vi "Non Delay Scheduler For Tardiness.vi"(8 "Number of  Jobs":i32=4, 9 "Number of Machines":i32=4, 10 "Processing Times":u16[][](array[numeric])=[[34, 15, 38, 95], [2, 89, 19, 7], [54, 70, 28, 34], [61, 9, 87, 29]], 11 "Schedule":u16[](array[numeric])=[12, 0, 7, 2, 6, 3, 13, 5, 1, 4, 14, 11, 10, 15, 8, 9]) -> (0 "Scheduled Jobs Order":u16[](array[numeric]), 1 "Job Completion Times":u16[](array[numeric]), 2 "Completion Times":u16[][](array[numeric]), 3 "Start Times":u16[][](array[numeric]), 4 "Machine Completion Times":u16[](array[numeric]))   [LabVIEW 2013, in "Scheduler.lvclass"]
uses:
  Scheduler.lvclass
  Priority Rule for ND Tardiness Engine.ctl
panel:
  out "Indices":i32[](array[numeric])
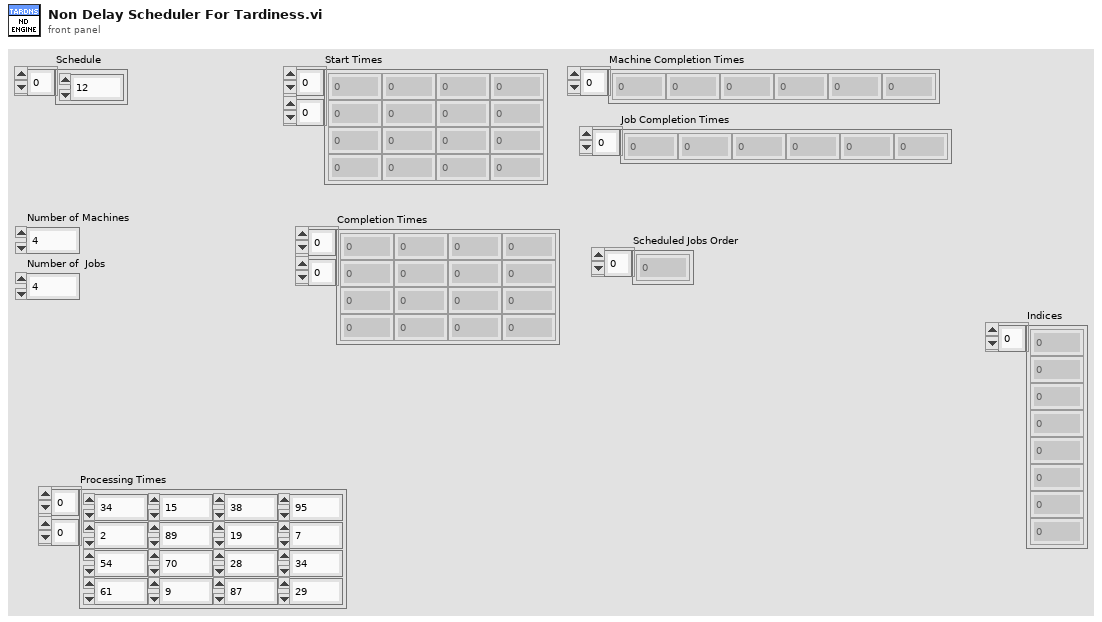
[diagram p1: front panel]
types:
  T1 = typedef "Scheduler.lvclass/Priority Rule for ND Tardiness Engine.ctl" = enum16{"SPT", "MST", "MDD"}
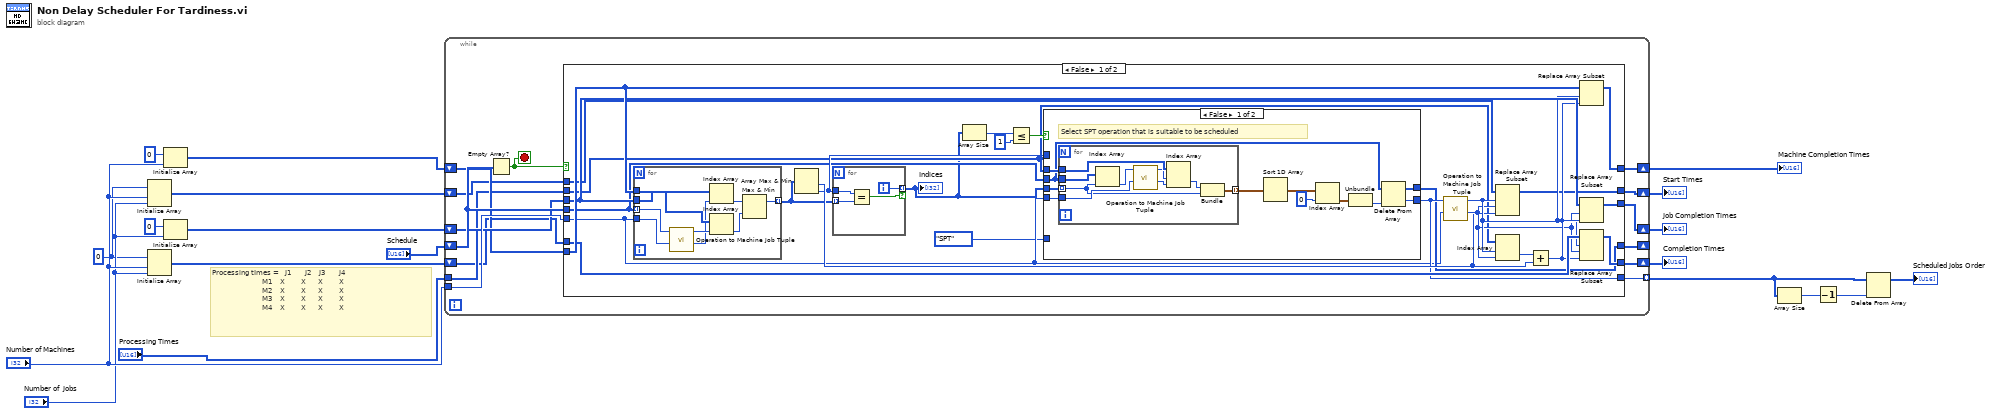
[diagram p0: block diagram]
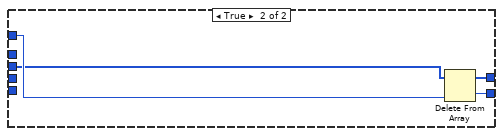
[diagram p2: hidden frame]
diagram:
  w3 = u16 0 ("element")
  # "Processing tImes =   J1       J2    J3       J4   \n                         M1    X        X      X        X\n                         M2    X        X      X        X\n                         M3    X        X      X        X\n                         M4    X        X      X        X"
  n1 = Initialize Array(w3, "Number of Machines", "Number of  Jobs") -> (w2:u16[][])
  n2 = Initialize Array(w3, "Number of Machines", "Number of  Jobs") -> (w14:u16[][])
  n3 = Initialize Array(u16 0 ("element"), "Number of Machines") -> (w16:u16[])
  n4 = Initialize Array(u16 0 ("element"), "Number of  Jobs") -> (w17:u16[])
  n5 = while {
    shift-right: [w25] -> _
    shift-left: "Schedule" -> [w32]
    tunnel: "Number of Machines" -> [w31]
    shift-right: [w28] -> w12
    shift-left: w17 -> [w30]
    shift-right: [w27] -> w11
    shift-left: w16 -> [w29]
    shift-right: [w23] -> w13
    shift-left: w14 -> [w24]
    tunnel: "Processing Times" -> [w26]
    tunnel: [w22] -> w9 mode=indexing
    shift-right: [w20] -> w1
    shift-left: w2 -> [w21]
    stop <- w33 stop-if-true
    n6 = Empty Array?(array=w32) -> (empty?=w33:bool)
    n7 = case shown="False" w33 {
      tunnel: w32 -> [w40 w98]
      tunnel: w31 -> [w35 _]
      tunnel: w30 -> [w57 w100]
      tunnel: w29 -> [w58 w99]
      tunnel: [w56 w100] -> w28
      tunnel: [w55 w99] -> w27
      tunnel: w26 -> [w37 _]
      tunnel: [w38 w98] -> w25
      tunnel: w24 -> [w54 w97]
      tunnel: [w53 w97] -> w23
      tunnel: [w39 _] -> w22
      tunnel: w21 -> [w50 w96]
      tunnel: [w46 w96] -> w20
      frame False {
        n8 = for {
          tunnel: w40 -> [w95] mode=indexing
          tunnel: w35 -> [w94]
          tunnel: w57 -> [w91]
          tunnel: w58 -> [w93]
          tunnel: [w87] -> w45 mode=indexing
          n9 = call "Operation to Machine Job Tuple.vi"("Number of Machines"=w94, "Operation Number"=w95) -> ("Job No"=w90:i32, "Machine No"=w92:i32)  [unwired: 8 in]
          n10 = Index Array(array=w91, index=w90) -> (element=w89:u16)
          n11 = Index Array(array=w93, index=w92) -> (element=w88:u16)
          n12 = Max & Min(x=w89, y=w88) -> (max(x,y)=w87:u16)  [unwired: 1 out]
        }
        n13 = Array Max & Min(array=w45) -> (min value=w47:u16, min index (indices)=w41:i32)  [unwired: 2 out]
        n14 = for {
          tunnel: w45 -> [w86] mode=indexing
          tunnel: w41 -> [w85]
          tunnel: [w84] -> w36 mode=indexing if=w83
          i -> [w84]
          n15 = Equal?(x=w85, y=w86) -> (x = y?=w83:bool)
        }
        "Indices" <- w36
        n16 = Array Size(array=w36) -> (size(s)=w44:i32)
        n17 = Less Or Equal?(x=w44, y=1) -> (x <= y?=w42:bool)
        n18 = case shown="False" w42 {
          tunnel: w41 -> [_ w82]
          tunnel: w40 -> [w62 w81]
          tunnel: [w59 w80] -> w38
          tunnel: [w60 w79] -> w39
          tunnel: w37 -> [w67 _]
          tunnel: w36 -> [w69 _]
          tunnel: w35 -> [w68 _]
          tunnel: Priority_Rule_for_ND_Tardiness_Engine."SPT" -> [_ _]
          frame False {
            # "Select SPT operation that is suitable to be scheduled"
            n19 = for {
              tunnel: w69 -> [w72] mode=indexing
              tunnel: w62 -> [w78]
              tunnel: w68 -> [w77]
              tunnel: w67 -> [w76]
              tunnel: [w71] -> w66 mode=indexing
              n20 = Index Array(array=w78, index=w72) -> (element=w70:u16)
              n21 = call "Operation to Machine Job Tuple.vi"("Number of Machines"=w77, "Operation Number"=w70) -> ("Job No"=w74:i32, "Machine No"=w75:i32)  [unwired: 8 in]
              n22 = Index Array(array=w76, index (row)=w75, index (col)=w74) -> (element=w73:u16)
              n23 = Bundle("Numeric"=w73, w72) -> (w71:cluster{"Numeric":u16, i32})  [unwired: 1 in]
            }
            n24 = Sort 1D Array(array=w66) -> (sorted array=w65:cluster{"Numeric":u16, i32}[])
            n25 = Index Array(array=w65, index=0) -> (element=w63:cluster{"Numeric":u16, i32})
            n26 = Unbundle(w63) -> (w61:i32)  [unwired: 1 out]
            n27 = Delete From Array(array=w62, index=w61) -> (deleted portion=w60:u16, array with subset deleted=w59:u16[])  [unwired: 1 in]
          }
          frame True {
            n28 = Delete From Array(array=w81, index=w82) -> (deleted portion=w79:u16, array with subset deleted=w80:u16[])  [unwired: 1 in]
          }
        }
        n29 = call "Operation to Machine Job Tuple.vi"("Number of Machines"=w35, "Operation Number"=w39) -> ("Job No"=w48:i32, "Machine No"=w49:i32)  [unwired: 8 in]
        n30 = Replace Array Subset(array=w50, new element=w47, index (row)=w49, index (col)=w48) -> (w46:u16[][])
        n31 = Index Array(array=w37, index (row)=w49, index (col)=w48) -> (element=w52:u16)
        n32 = Add(x=w52, y=w47) -> (x+y=w51:u16)
        n33 = Replace Array Subset(array=w58, new element=w51, index=w49) -> (w55:u16[])
        n34 = Replace Array Subset(array=w57, new element=w51, index=w48) -> (w56:u16[])
        n35 = Replace Array Subset(array=w54, new element=w51, index (row)=w49, index (col)=w48) -> (w53:u16[][])
      }
      frame True {
      }
    }
  }
  "Completion Times" <- w13
  "Job Completion Times" <- w12
  "Machine Completion Times" <- w11
  "Start Times" <- w1
  n36 = Array Size(array=w9) -> (size(s)=w8:i32)
  n37 = Decrement(x=w8) -> (x-1=w7:i32)
  n38 = Delete From Array(array=w9, index=w7) -> (array with subset deleted=→"Scheduled Jobs Order":u16[])  [unwired: 1 in, 1 out]
